vi "Encoder SubVI.vi"(10 "Reset Encoders":bool) -> (0 "error out":errorcluster, 1 "Distance M2":dbl, 2 "Distance M1":dbl, 3 "Distance M0":dbl)   [LabVIEW 2018]
uses:
  <vilib>/Studica/Studica Toolkit/Background/Mxp Selection.ctl
panel:
  in  "stop":bool
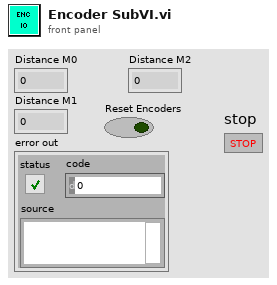
[diagram p1: front panel]
types:
  T1 = typedef "Mxp Selection.ctl" = enum16{"MXP A", "MXP B"}
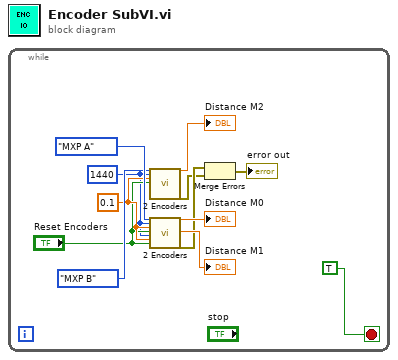
[diagram p0: block diagram]
diagram:
  n1 = while {
    stop <- TRUE stop-if-true
    w3 = u32 1440 ("Ticks Per Rev M0")
    w8 = 0.1 ("Wheel Diameter M0 (inches)")
    n2 = call <vilib>:"2 Encoders.vi"("Mxp Side"=Mxp_Selection."MXP B", "Ticks Per Rev M0"=w3, "Wheel Diameter M0 (inches)"=w8, "Reset Encoder 0"="Reset Encoders") -> ("Distance M0 (inches)"=→"Distance M2":dbl, "error out"=w5:errorcluster)  [unwired: 21 in, 1 out]
    n3 = call <vilib>:"2 Encoders.vi"("Mxp Side"=Mxp_Selection."MXP A", "Ticks Per Rev M0"=w3, "Wheel Diameter M0 (inches)"=w8, "Reset Encoder 0"="Reset Encoders", "Ticks Per Rev M1"=w3, "Wheel Diameter M1 (inches)"=w8, "Reset Encoder 1"="Reset Encoders") -> ("Distance M0 (inches)"=→"Distance M0":dbl, "Distance M1 (inches)"=→"Distance M1":dbl, "error out"=w6:errorcluster)  [unwired: 18 in]
    n4 = Merge Errors(w6, w5) -> (→"error out":errorcluster)
  }
